vi "Read TestType.vi"(8 "error in (no error)":errorcluster, 11 "TestSeqClass in":refnum<class "TestSeqClass.lvclass">) -> (0 "error out":errorcluster, 2 "TestType":T1, 3 "TestSeqClass out":refnum<class "TestSeqClass.lvclass">)   [LabVIEW 2019, in "TestSeqClass.lvclass"]
uses:
  TestSeqClass.lvclass
  Typedef/TestTypeSelect.ctl
  TestSeqClass.lvclass/TestSeqClass.ctl
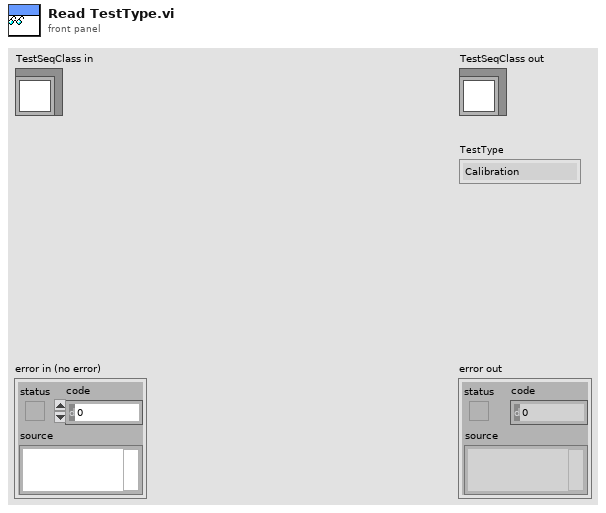
[diagram p1: front panel]
types:
  T1 = typedef "TestTypeSelect.ctl" = enum16{"Calibration", "Testing"}
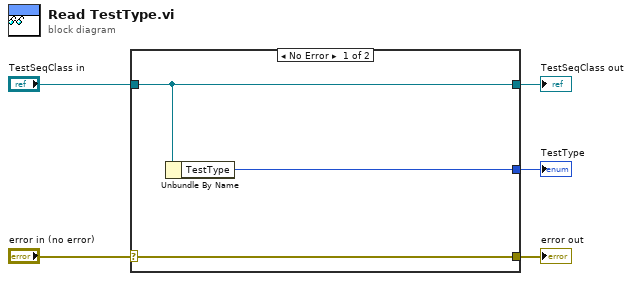
[diagram p0: block diagram]
diagram:
  n1 = case shown="No Error" "error in (no error)" {
    selector: "error in (no error)" -> [w8 w9]
    tunnel: [w8 w9] -> w4
    tunnel: [w7 w10] -> w2
    tunnel: "TestSeqClass in" -> [w7 w10]
    tunnel: [w6 _] -> w1
    frame No Error {
      n2 = Unbundle By Name(w7) -> ("TestType"=w6:T1)
    }
    frame Error {
    }
  }
  "error out" <- w4
  "TestSeqClass out" <- w2
  "TestType" <- w1
